vi "gun_rt_fast_downstream_datastore.vi"(10 "data_store_mode":enum16{"Set", "Get"}(ring), 11 "gun_rt_fast_downstream_data":T1) -> (3 "gun_rt_fast_downstream_data out":T1)   [LabVIEW 2011]
uses:
  gun_rt_fast_downstream_data.ctl
  gun_motor_state.ctl
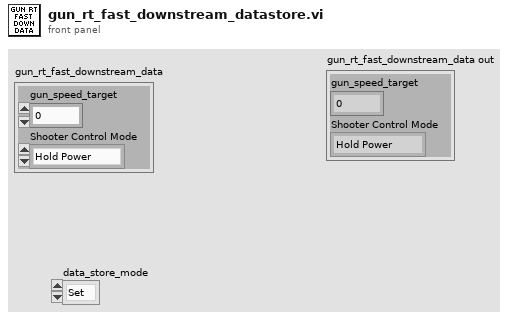
[diagram p1: front panel]
types:
  T1 = typedef "gun_rt_fast_downstream_data.ctl" = cluster{"gun_speed_target":dbl, "Shooter Control Mode":T2}
  T2 = typedef "gun_motor_state.ctl" = enum16{"Hold Power", "Hold Speed", "Hold Distance", "Stop"}
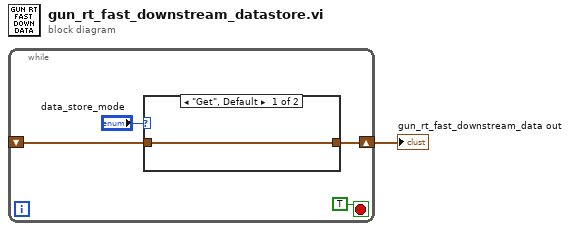
[diagram p0: block diagram]
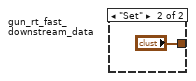
[diagram p2: hidden frame]
diagram:
  n1 = while {
    shift-right: [w3] -> w1
    shift-left: _ -> [w2]
    stop <- TRUE stop-if-true
    n2 = case shown="\"Get\", Default" "data_store_mode" {
      tunnel: [w6 "gun_rt_fast_downstream_data"] -> w3
      tunnel: w2 -> [w6 _]
      frame "Get", Default {
      }
      frame "Set" {
      }
    }
  }
  "gun_rt_fast_downstream_data out" <- w1
